vi "Build XY Graph.vi"(9 "Meas Temp":dbl[](array[numeric]), 10 "Meas Time":timestamp[](array[timestamp]), 11 "XY In":cluster{timestamp[], "Y":dbl[]}[](array[cluster])) -> (3 "XY out":cluster{timestamp[], "Y":dbl[]}[](array[cluster]))   [LabVIEW 2021]
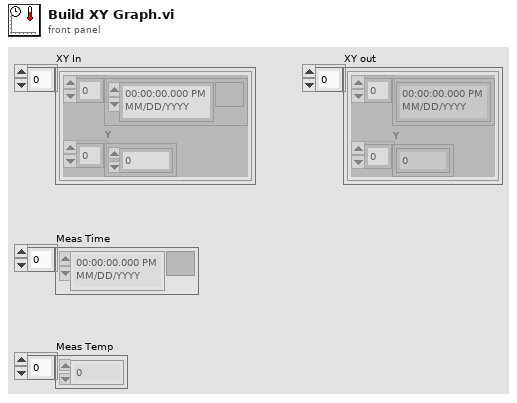
[diagram p1: front panel]
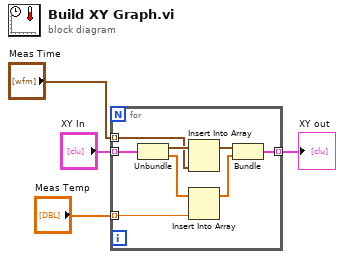
[diagram p0: block diagram]
diagram:
  n1 = for {
    tunnel: "Meas Time" -> [w9] mode=indexing
    tunnel: "Meas Temp" -> [w7] mode=indexing
    tunnel: [w12] -> w2 mode=indexing
    tunnel: "XY In" -> [w11] mode=indexing
    n2 = Unbundle(w11) -> (w10:timestamp[], "Y"=w8:dbl[])
    n3 = Insert Into Array(array=w10, new element=w9) -> (w6:timestamp[])  [unwired: 1 in]
    n4 = Insert Into Array(array=w8, new element=w7) -> (w5:dbl[])  [unwired: 1 in]
    n5 = Bundle(w6, "Y"=w5) -> (w12:cluster{timestamp[], "Y":dbl[]})  [unwired: 1 in]
  }
  "XY out" <- w2
